vi "FROG_ReadFromFile.vi"(5 "File Path":path) -> (0 "Delay Info":T1, 1 "Spectrum Info":T2, 2 "Experiment Trace":dbl[][](array[numeric]))   [LabVIEW 2013]
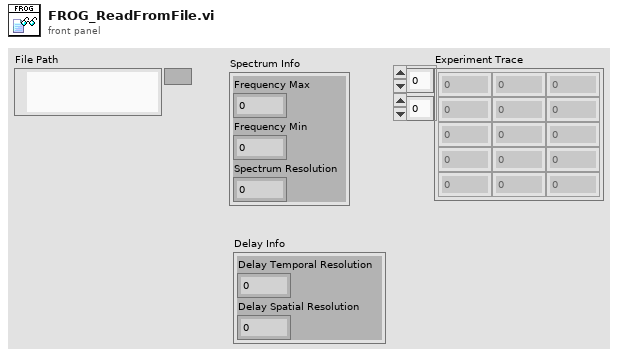
[diagram p1: front panel]
types:
  T1 = cluster{"Delay Temporal Resolution":u16, "Delay Spatial Resolution":u16}
  T2 = cluster{"Frequency Max":dbl, "Frequency Min":dbl, "Spectrum Resolution":u16}
  T3 = cluster{"Temporal Resolution":u16, "Spatial Resolution (nm)":u16}
  T4 = cluster{"Wavelength Max (nm)":dbl, "Wavelength Min (nm)":dbl, "Spectrum Resolution":u16}
  T5 = cluster{"Frequency Max (G-rad/s)":dbl, "Frequency Min (G-rad/s)":dbl, "Spectrum Resolution":u16}
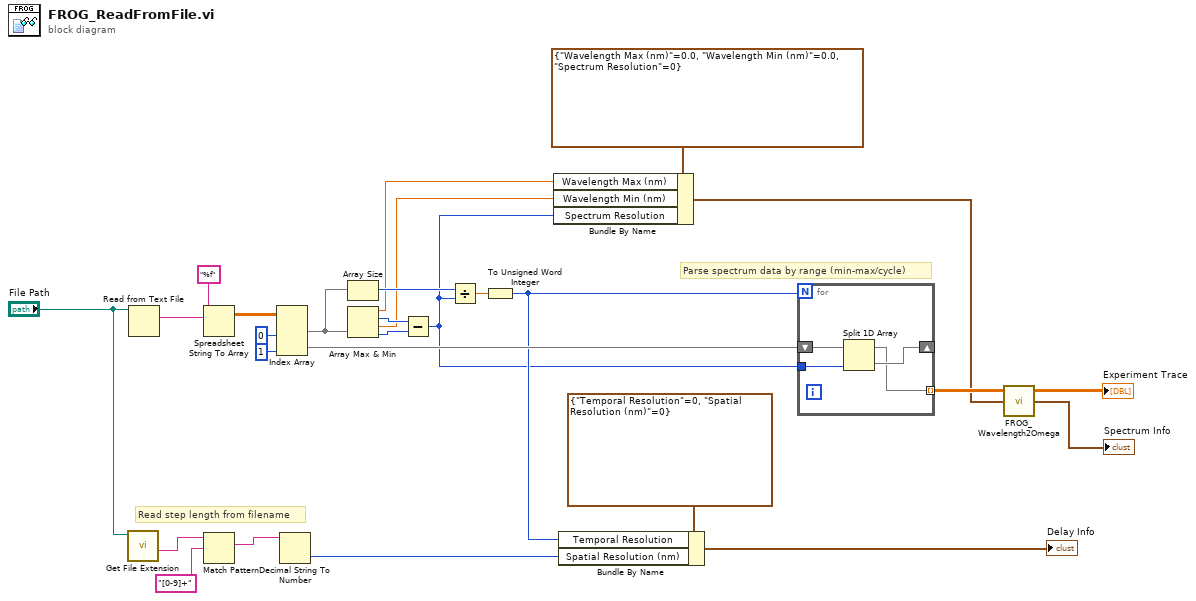
[diagram p0: block diagram]
diagram:
  # "Read step length from filename"
  # "Parse spectrum data by range (min-max/cycle)"
  n1 = call <vilib>:"Get File Extension.vi"("file"="File Path") -> ("filename without extension"=w14:string)  [unwired: 7 in, 3 out]
  n2 = Read from Text File(file (use dialog)="File Path") -> (text=w18:string)  [unwired: 3 in, 3 out]
  n3 = Spreadsheet String To Array(format string="%f", spreadsheet string=w18) -> (array=w20:dbl[][])  [unwired: 2 in]
  n4 = Match Pattern(string=w14, regular expression="[0-9]+") -> (match substring=w12:string)  [unwired: 1 in, 3 out]
  n5 = Index Array(array=w20, index (col) #1=0 ("disabled index (col)"), index (col) #2=1 ("index (col)")) -> (element #1=w23:dbl[], element #2=w24:dbl[])  [unwired: 2 in]
  n6 = Decimal String To Number(string=w12) -> (number=w5:i32)  [unwired: 2 in, 1 out]
  n7 = Array Size(array=w23) -> (size(s)=w27:i32)
  n8 = Array Max & Min(array=w23) -> (max value=w8:dbl, max index (indices)=w25:i32, min value=w7:dbl, min index (indices)=w26:i32)
  n9 = Subtract(x=w25, y=w26) -> (x-y=w9:i32)
  n10 = Divide(x=w27, y=w9) -> (x/y=w17:dbl)
  n11 = To Unsigned Word Integer(number=w17) -> (unsigned 16bit integer=w10:u16)
  n12 = Bundle By Name(cluster=T4 {"Wavelength Max (nm)"=0.0, "Wavelength Min (nm)"=0.0, "Spectrum Resolution"=0}, "Wavelength Max (nm)"=w8, "Wavelength Min (nm)"=w7, "Spectrum Resolution"=w9) -> (w1:T4)
  n13 = Bundle By Name(cluster=T3 {"Temporal Resolution"=0, "Spatial Resolution (nm)"=0}, "Temporal Resolution"=w10, "Spatial Resolution (nm)"=w5) -> (→"Delay Info":T3)
  n14 = for {
    N: w10 -> [_]
    shift-right: [w30] -> _
    shift-left: w24 -> [w31]
    tunnel: [w29] -> w4 mode=indexing
    tunnel: w9 -> [w28]
    n15 = Split 1D Array(array=w31, index=w28) -> (first subarray=w29:dbl[], second subarray=w30:dbl[])
  }
  n16 = call "FROG_Wavelength2Omega.vi"("Spectrum Info"=w1, "Experiment Trace"=w4) -> ("Spectrum Info"=→"Spectrum Info":T5, "Converted Trace"=→"Experiment Trace":dbl[][])  [unwired: 2 in]
